vi "uTTA_QualifiyResponse.vi"(4 "error in":errorcluster, 5 "Response Qualifier(\"\")":string, 6 "RX Termination(\\n)":string="\n", 7 "Databuffer IN":string) -> (0 "error out":errorcluster, 1 "Response":string, 2 "Found response":bool, 3 "DataBuffer out":string)   [LabVIEW 2021]
panel:
  out "size(s)":i32
  out "Array of Strings":string[](array[string])
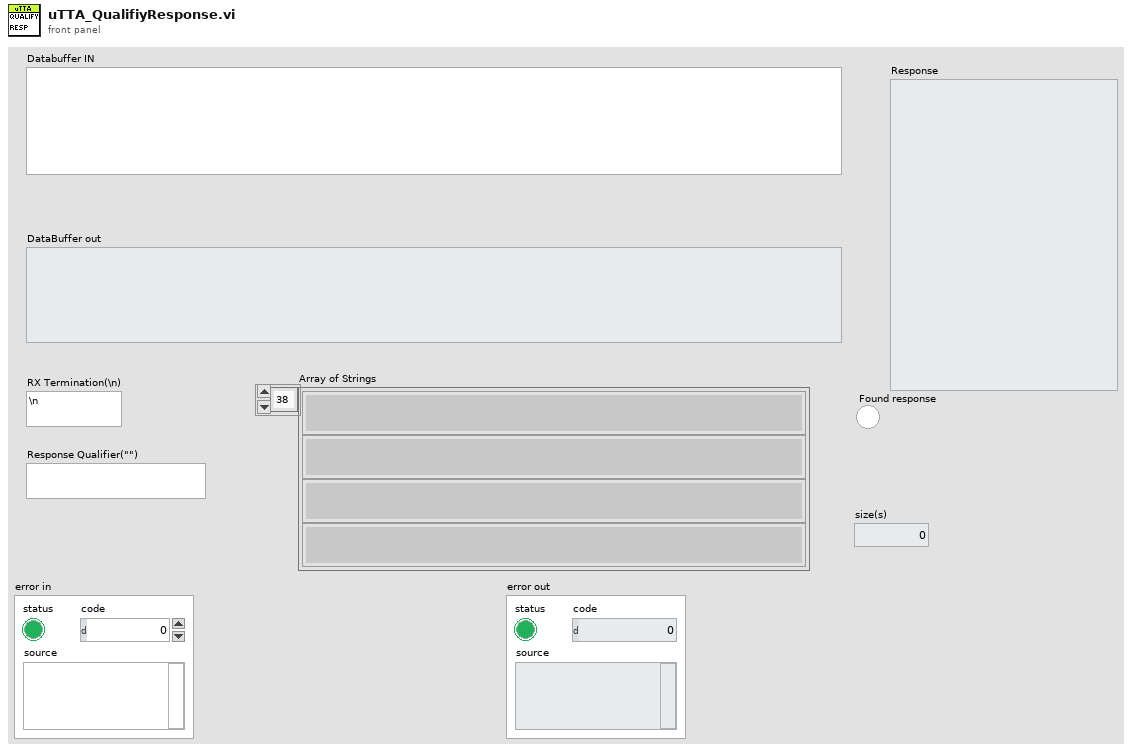
[diagram p1: front panel]
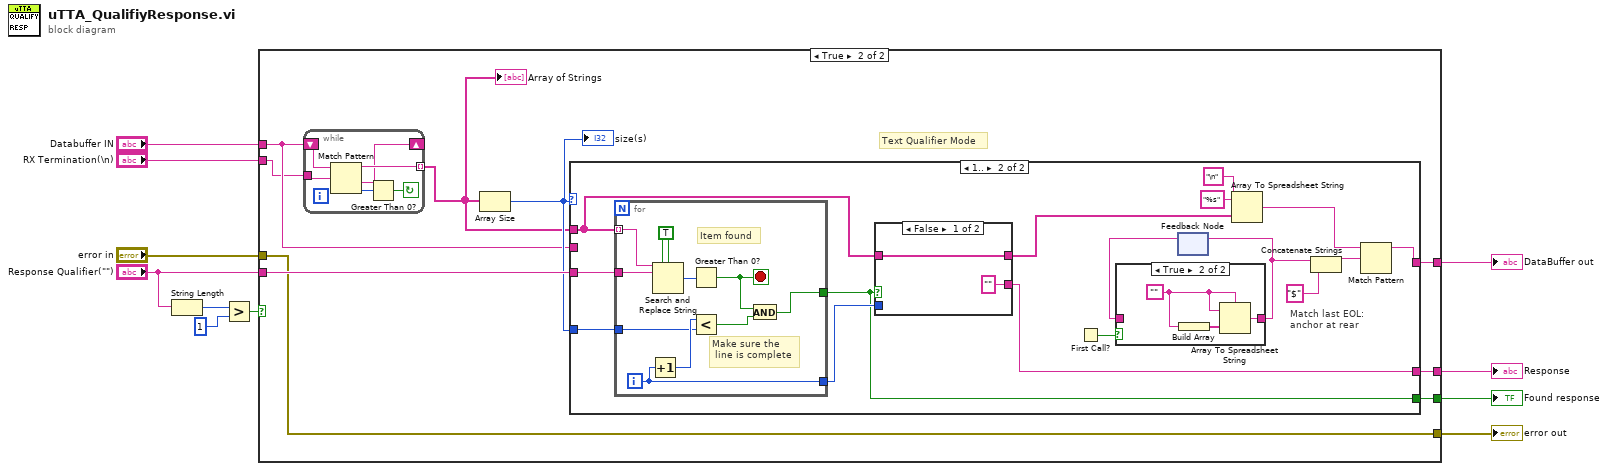
[diagram p0: block diagram]
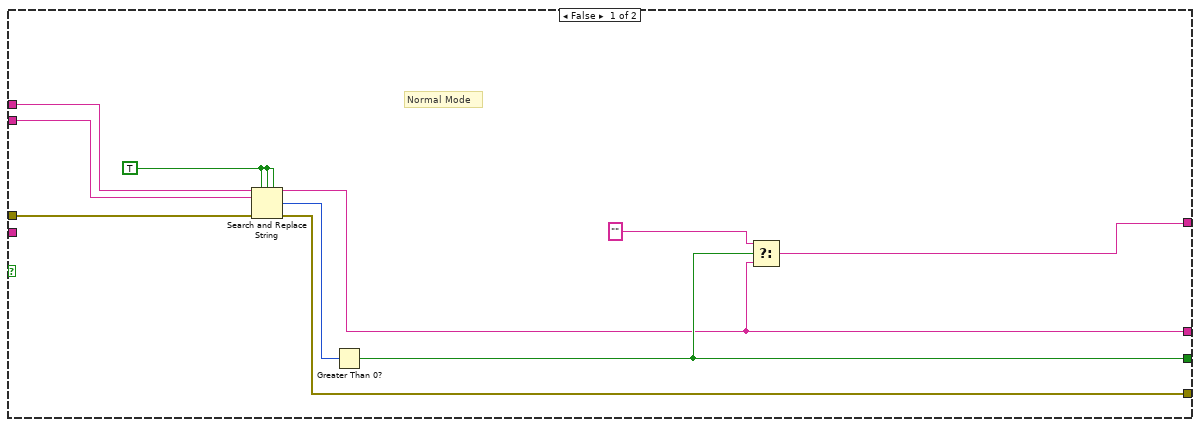
[diagram p2: hidden frame]
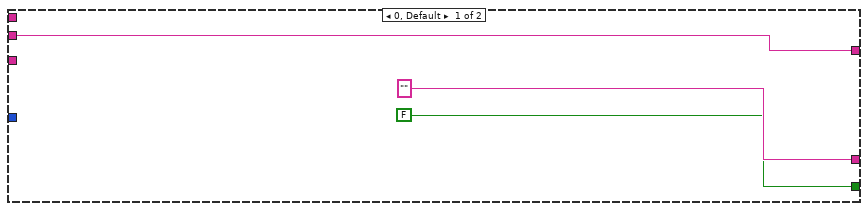
[diagram p3: hidden frame]
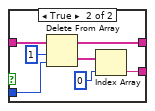
[diagram p5: hidden frame]
diagram:
  n1 = String Length(string="Response Qualifier(\"\")") -> (length=w3:i32)
  n2 = Greater?(x=w3, y=1) -> (0:w2:bool)
  n3 = case shown="True" w2 {
    tunnel: "Response Qualifier(\"\")" -> [_ w30]
    tunnel: [w13 w29] -> w10
    tunnel: "Databuffer IN" -> [w18 w23]
    tunnel: [w14 w28] -> w9
    tunnel: [w16 w27] -> w11
    tunnel: "RX Termination(\\n)" -> [w21 w22]
    tunnel: "error in" -> [w20 w26]
    tunnel: [w19 w26] -> w8
    frame False {
      w12 = TRUE ("ignore case? (F)")
      # "Normal Mode"
      n4 = Search and Replace String(replace all?=w12, case sensitive?=w12, multiline?=w12, input string=w18, search string=w21, error in=w20) -> (result string=w14:string, number of replacements=w17:i32, error out=w19:errorcluster)  [unwired: 2 in, 1 out]
      n5 = Greater Than 0?(x=w17) -> (x > 0?=w16:bool)
      n6 = Select(t="" ("delimited string"), s=w16, f=w14) -> (s? t:f=w13:string)
    }
    frame True {
      # "Text Qualifier Mode"
      n7 = while {
        tunnel: w22 -> [w35]
        tunnel: [w34] -> w24 mode=indexing
        shift-right: [w33] -> _
        shift-left: w23 -> [w36]
        stop <- w31 continue-if-true
        n8 = Match Pattern(string=w36, regular expression=w35) -> (before substring=w34:string, after substring=w33:string, offset past match=w32:i32)  [unwired: 1 in, 1 out]
        n9 = Greater Than 0?(x=w32) -> (x > 0?=w31:bool)
      }
      "Array of Strings" <- w24
      n10 = Array Size(array=w24) -> (size(s)=w25:i32)
      "size(s)" <- w25
      n11 = case shown="1.." w25 {
        tunnel: w30 -> [_ w55]
        tunnel: [w39 w45] -> w29
        tunnel: w24 -> [_ w53]
        tunnel: w23 -> [w39 _]
        tunnel: ["" w52] -> w28
        tunnel: [FALSE w51] -> w27
        tunnel: w25 -> [_ w50]
        frame 0, Default {
        }
        frame 1.. {
          # "Match last EOL:\nanchor at rear"
          n12 = for {
            tunnel: w53 -> [w67] mode=indexing
            tunnel: w55 -> [w68]
            tunnel: [w64] -> w51
            tunnel: [w63] -> w54
            tunnel: w50 -> [w61]
            i -> [w63]
            stop <- w65 stop-if-true
            w69 = TRUE ("replace all? (F)")
            # "Make sure the\n line is complete"
            # "Item found"
            n13 = Increment(x=w63) -> (x+1=w62:i32)
            n14 = Search and Replace String(replace all?=w69, case sensitive?=w69, input string=w67, search string=w68) -> (number of replacements=w66:i32)  [unwired: 4 in, 3 out]
            n15 = Greater Than 0?(x=w66) -> (x > 0?=w65:bool)
            n16 = Less?(x=w62, y=w61) -> (x < y?=w60:bool)
            n17 = And(x=w65, y=w60) -> (x .and. y?=w64:bool)
          }
          n18 = case shown="False" w51 {
            tunnel: w54 -> [_ w76]
            tunnel: w53 -> [w71 w78]
            tunnel: [w71 w75] -> w43
            tunnel: ["" w72] -> w52
            frame False {
            }
            frame True {
              n19 = Delete From Array(array=w78, length=1, index=w76) -> (deleted portion=w74:string[], array with subset deleted=w75:string[])
              n20 = Index Array(array=w74, index=0) -> (element=w72:string)
            }
          }
          n21 = First Call?() -> (First Call?: T/F=w42:bool)
          n22 = feedback #1() -> (w41:string)  [unwired: 1 in]
          n23 = case shown="True" w42 {
            tunnel: [w56 w57] -> w40
            tunnel: w41 -> [w56 _]
            frame False {
            }
            frame True {
              w58 = "" ("Empty String\n(hidden on FP)")
              n24 = Build Array(w58) -> (w59:string[])
              n25 = Array To Spreadsheet String(delimiter (Tab)=w58, array=w59, 3:w58) -> (spreadsheet string=w57:string)
            }
          }
          n26 = feedback-in #1(w40) -> ()
          n27 = Array To Spreadsheet String(delimiter (Tab)="\n", array=w43, 3:"%s" ("format string")) -> (spreadsheet string=w49:string)
          n28 = Concatenate Strings(w40, "$" ("Substring")) -> (w48:string)
          n29 = Match Pattern(string=w49, regular expression=w48) -> (before substring=w45:string)  [unwired: 1 in, 3 out]
        }
      }
    }
  }
  "Found response" <- w11
  "DataBuffer out" <- w10
  "Response" <- w9
  "error out" <- w8
